vi "Periodic Tasks.vi"(8 "error in":errorcluster) -> ()   [LabVIEW 2015]
doc: "This VI runs in parallel to other tasks. It can contain as many user-defined periodic loops as you need. These can carry out PID or other sorts of timed response."
uses:
  <vilib>/Rock Robotics/WPI/DriverStation/WPI_DriverStationRobotMode2.ctl
  <vilib>/Rock Robotics/WPI/Utilities/WPI_GetSetVariantRefNum.vi
  Robot Global Data.vi
panel:
  in  "file path (use dialog)":path
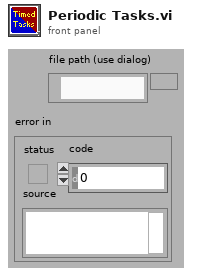
[diagram p1: front panel]
types:
  T1 = enum16{"open", "replace", "create", "open or create", "replace or create", "replace or create with confirmation"}
  T2 = typedef "WPI_JoystickDevRef.ctl" = cluster{"Device":T3}
  T3 = typedef "WPI_JoystickDeviceEnum.ctl" = enum16{"USB 0", "USB 1", "USB 2", "USB 3", "USB 4", "USB 5"}
  T4 = typedef "WPI_RobotDriveDevRef.ctl" = cluster{"DevStatus":errorcluster, "Motors[]":T5[], "Square Inputs":bool, "Max Output":dbl}
  T5 = typedef "WPI_MotorControlDeviceRef.ctl" = cluster{"DeviceStatus":errorcluster, "Type":T6, "PWM":cluster{"PWM Channel":T7, "DeadBand":T8}, "CAN":cluster{"Device Number":u8, "Control Mode":T9, "Semaphore":T10, "Max Vout":dbl, "TalonSRX Control Mode":T11}, "Invert":bool}
  T6 = typedef "WPI_MotorControlType.ctl" = enum16{"PWM", "CAN", "CANTalonSRX"}
  T7 = typedef "FPGA_DIOPWMChannel.ctl" = enum8{"PWM 0", "PWM 1", "PWM 2", "PWM 3", "PWM 4", "PWM 5", "PWM 6", "PWM 7", "PWM 8", "PWM 9", "PWM MXP 0", "PWM MXP 1", "PWM MXP 2", "PWM MXP 3", "PWM MXP 4", "PWM MXP 5", "PWM MXP 6", "PWM MXP 7", "PWM MXP 8", "PWM MXP 9", "Invalid"}
  T8 = typedef "WPI_PWMDeadband.ctl" = cluster{"Name":string, "maxPositivePwm":i32, "minPositivePwm":i32, "centerPwm":i32, "maxNegativePwm":i32, "minNegativePwm":i32, "angularRange":u16}
  T9 = typedef "WPI_CANJaguar_ControlMode.ctl" = enum8{"Percent VBus", "Current", "Speed", "Position", "Voltage"}
  T10 = typedef "Semaphore RefNum" = refnum<k1>
  T11 = typedef "WPI_CANTalonSRX_APIControlMode.ctl" = enum8{"Percent VBus", "Speed", "Position", "Slave", "Unchanged / Invalid", "Voltage Compensation", "Current", "Motion Profile"}
  T12 = cluster{"JoystickDevRef":T2, "RobotDriveDevRef":T4}
  T13 = typedef "WPI_DriverStationRobotMode2.ctl" = enum16{"Autonomous Disabled", "Autonomous Enabled", "Teleop Disabled", "Teleop Enabled", "Disconnected", "Finish", "Test Disabled", "Test Enabled", "Emergency Stopped"}
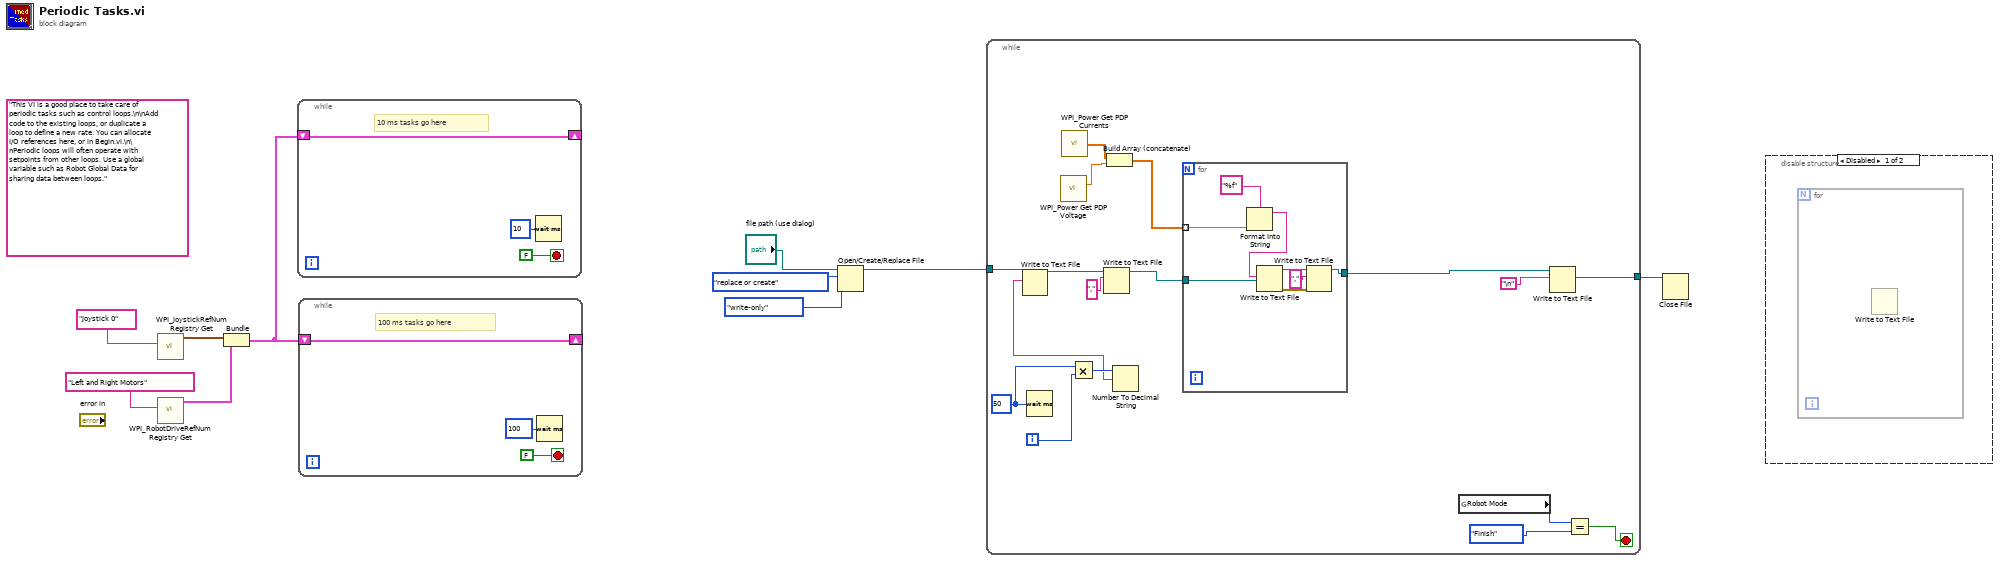
[diagram p0: block diagram]
diagram:
  (unwired) "This VI is a good place to take care of periodic tasks such as control loops.\n\nAdd code to the existing loops, or duplicate a loop to define a new rate. You can allocate I/O references here, or in Begin.vi.\n\nPeriodic loops will often operate with setpoints from other loops. Use a global variable such as Robot Global Data for sharing data between loops."
  n1 = call <vilib>:"WPI_JoystickRefNum Registry Get.vi"("refnum name"="Joystick 0") -> ("JoystickDevRef"=w8:T2)  [unwired: 1 in, 9 out]
  n2 = call <vilib>:"WPI_RobotDriveRefNum Registry Get.vi"("refnum name"="Left and Right Motors") -> ("RobotDriveDevRef"=w7:T4)  [unwired: 1 in, 9 out]
  n3 = Bundle("JoystickDevRef"=w8, "RobotDriveDevRef"=w7) -> (w6:T12)  [unwired: 1 out]
  n4 = while {
    shift-right: [w11] -> _
    shift-left: w6 -> [w11]
    stop <- FALSE stop-if-true
    # "10 ms tasks go here"
    n5 = Wait (ms)(milliseconds to wait=u32 10) -> ()  [unwired: 1 out]
  }
  n6 = while {
    shift-right: [w14] -> _
    shift-left: w6 -> [w14]
    stop <- FALSE stop-if-true
    # "100 ms tasks go here"
    n7 = Wait (ms)(milliseconds to wait=u32 100) -> ()  [unwired: 1 out]
  }
  n8 = Open/Create/Replace File(file path (use dialog)="file path (use dialog)", operation (0:open)=T1."replace or create", access (0:read/write)=enum16{"read/write", "read-only", "write-only"}."write-only") -> (refnum out=w2:refnum<file>)  [unwired: 3 in, 2 out]
  n9 = while {
    tunnel: w2 -> [w33]
    tunnel: [w23] -> w1
    i -> [w31]
    stop <- w17 stop-if-true
    w32 = u32 50 ("milliseconds to wait")
    n10 = Wait (ms)(milliseconds to wait=w32) -> ()  [unwired: 1 out]
    n11 = call <vilib>:"WPI_Power Get PDP Voltage.vi"() -> ("voltage (V)"=w21:dbl)  [unwired: 14 in, 1 out]
    n12 = call <vilib>:"WPI_Power Get PDP Currents.vi"() -> ("all currents (A)"=w22:dbl[])  [unwired: 13 in, 2 out]
    n13 = Multiply(x=w32, y=w31) -> (x*y=w30:u32)
    n14 = Build Array (concatenate)(w22, w21) -> (w20:dbl[])
    n15 = Number To Decimal String(number=w30) -> (decimal integer string=w29:string)  [unwired: 1 in]
    n16 = Write to Text File(file (use dialog)=w33, text=w29) -> (refnum out=w28:refnum<file>)  [unwired: 2 in, 2 out]
    n17 = Write to Text File(file (use dialog)=w28, text=",") -> (refnum out=w27:refnum<file>)  [unwired: 2 in, 2 out]
    n18 = for {
      tunnel: w27 -> [w41]
      tunnel: [w35] -> w25
      tunnel: w20 -> [w34] mode=indexing
      n19 = Format Into String(format string="%f", w34) -> (resulting string=w39:string)  [unwired: 2 in, 1 out]
      n20 = Write to Text File(file (use dialog)=w41, text=w39) -> (refnum out=w37:refnum<file>, error out=w38:errorcluster)  [unwired: 2 in, 1 out]
      n21 = Write to Text File(file (use dialog)=w37, text=",", error in=w38) -> (refnum out=w35:refnum<file>)  [unwired: 1 in, 2 out]
    }
    n22 = global read "Robot Global Data.vi" "Robot Mode"() -> (w19:T13)
    n23 = Write to Text File(file (use dialog)=w25, text="\n") -> (refnum out=w23:refnum<file>)  [unwired: 2 in, 2 out]
    n24 = Equal?(x=w19, y=WPI_DriverStationRobotMode2."Finish" ("Robot Mode")) -> (x = y?=w17:bool)
  }
  n25 = Close File(refnum=w1) -> ()  [unwired: 1 in, 2 out]
  n26 = disable-structure shown="Disabled" {
    frame Disabled {
      n27 = for {
        n28 = Write to Text File() -> ()  [unwired: 4 in, 3 out]
      }
    }
    frame Enabled {
    }
  }
